vi "Stop Button FGV.vi"(7 "Operation":enum16{"GET", "SET"}(ring), 11 "Stop Button":bool) -> (3 "Stop ButtonOut":bool)   [LabVIEW 2014]
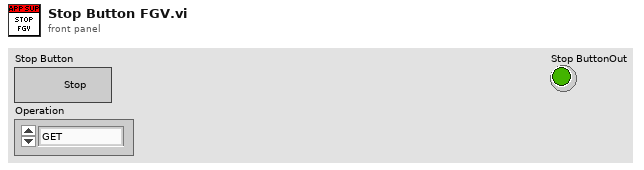
[diagram p1: front panel]
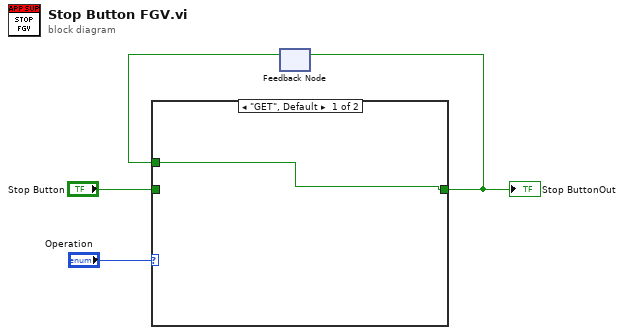
[diagram p0: block diagram]
diagram:
  n1 = feedback #1() -> (w1:bool)  [unwired: 1 in]
  n2 = case shown="\"GET\", Default" "Operation" {
    tunnel: [w5 w6] -> w2
    tunnel: "Stop Button" -> [_ w6]
    tunnel: w1 -> [w5 _]
    frame "GET", Default {
    }
    frame "SET" {
    }
  }
  "Stop ButtonOut" <- w2
  n3 = feedback-in #1(w2) -> ()
